vi "Stop Acquisition.vi"(8 "error in (no error)":errorcluster, 11 "Hardware Resources in":T1={"DO"={"task name"="AI", "task_ref"="", "lines"=""}}) -> (0 "error out":errorcluster)   [LabVIEW 2014, in "PLS Digital Control.lvlib"]
doc: "Stops the acquisition."
uses:
  PLS Digital Control.lvlib
  Hardware Configuration.ctl
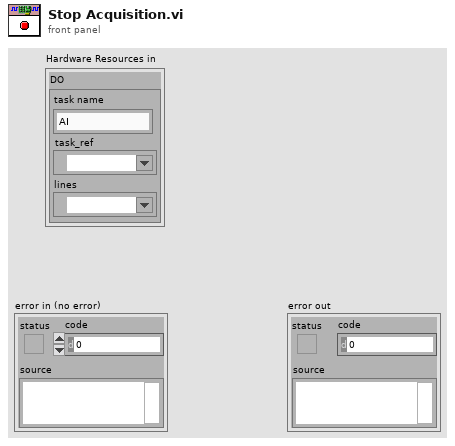
[diagram p1: front panel]
types:
  T1 = typedef "PLS Digital Control.lvlib/Hardware Configuration.ctl" = cluster{"DO":cluster{"task name":string, "task_ref":refnum<k21>, "lines":tag}}
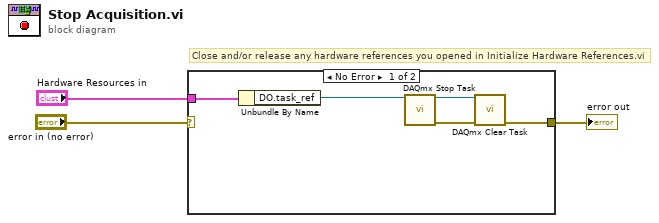
[diagram p0: block diagram]
diagram:
  # "Close and/or release any hardware references you opened in Initialize Hardware References.vi"
  n1 = case shown="No Error" "error in (no error)" {
    selector: "error in (no error)" -> [_ w9]
    tunnel: [w4 w9] -> w2
    tunnel: "Hardware Resources in" -> [w8 _]
    frame No Error {
      n2 = Unbundle By Name(w8) -> ("DO.task_ref"=w7:refnum<k21>)
      n3 = call <vilib>:"DAQmx Stop Task.vi"("task/channels in"=w7) -> ("task out"=w6:refnum<k21>, "error out"=w5:errorcluster)  [unwired: 13 in]
      n4 = call <vilib>:"DAQmx Clear Task.vi"("task in"=w6, "error in"=w5) -> ("error out"=w4:errorcluster)  [unwired: 13 in]
    }
    frame Error {
    }
  }
  "error out" <- w2
